vi "Pre Launch Init.vi"(11 "Actor 1 - State machine in":refnum<class "Actor 1 - State machine.lvclass">) -> (0 "error out":errorcluster, 3 "Actor 1 - State machine out":refnum<class "Actor 1 - State machine.lvclass">)   [LabVIEW 2020, in "Actor 1 - State machine.lvlib" / "Actor 1 - State machine.lvclass"]
doc: "(<B>Filename</B>: Actor Framework.lvlib:Actor.lvclass:Pre Launch Init.vi)\n\nDefines behavior that occurs after the Launch Nested Actor method is invoked but before the actor's Actor Core method begins running.\n\nBy default, this method does nothing. A descendant class may override it to define behavior."
uses:
  Actor 1 - State machine.lvclass
  Actor 1 - State machine.lvclass/Actor 1 - State machine.ctl
  <vilib>/ActorFramework/Actor/Actor.lvclass
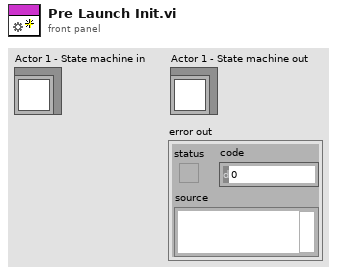
[diagram p1: front panel]
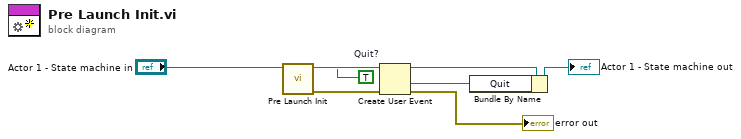
[diagram p0: block diagram]
diagram:
  w5 = TRUE  # Quit?
  n1 = call-parent "Pre Launch Init.vi"("Actor in"="Actor 1 - State machine in") -> ("error out"=w4:errorcluster, "Actor out"=w7:refnum<class "Actor 1 - State machine.lvclass">)  [unwired: 9 in]
  n2 = Create User Event(user event datatype=w5, error in=w4) -> (user event=w1:refnum<user-event>, error out=→"error out":errorcluster)
  n3 = Bundle By Name(cluster=w7, "Quit"=w1) -> (→"Actor 1 - State machine out":refnum<class "Actor 1 - State machine.lvclass">)
